vi "LVClass_SlopesPostProcessList Write SlopesPostProccessor  ptr create.vi"(8 "error in (no error)":errorcluster, 10 "Enum":T1, 11 "SlopesPostProcessorList in":refnum<class "SlopesPostProcessorList.lvclass">) -> (0 "error out":errorcluster, 3 "SlopesPostProcessorList out":refnum<class "SlopesPostProcessorList.lvclass">)   [LabVIEW 2020, in "SlopesPostProcessorList.lvclass"]
uses:
  SlopesPostProcessorList.lvclass
  Controls/Handle creation.ctl
  SlopesPostProcessorList.lvclass/SlopesPostProcessorList.ctl
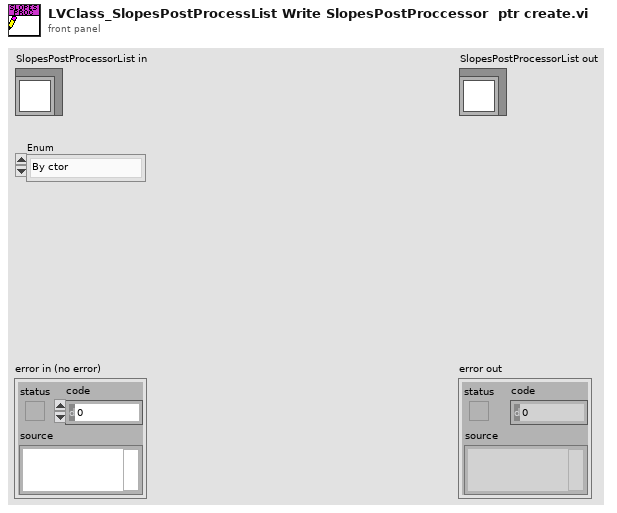
[diagram p1: front panel]
types:
  T1 = typedef "Handle creation.ctl" = enum16{"By ctor", "By write function"}
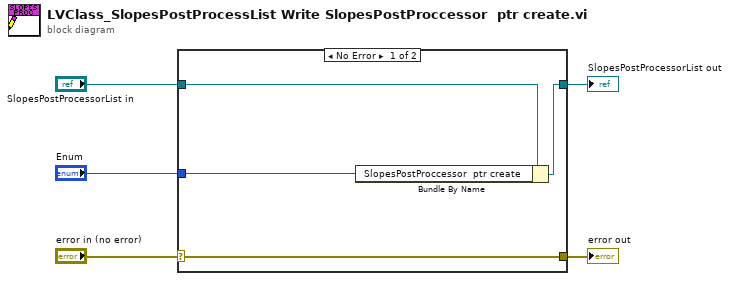
[diagram p0: block diagram]
diagram:
  n1 = case shown="No Error" "error in (no error)" {
    selector: "error in (no error)" -> [w9 w10]
    tunnel: [w9 w10] -> w4
    tunnel: [w7 w11] -> w2
    tunnel: "SlopesPostProcessorList in" -> [w8 w11]
    tunnel: "Enum" -> [w6 _]
    frame No Error {
      n2 = Bundle By Name(cluster=w8, "SlopesPostProccessor  ptr create"=w6) -> (w7:refnum<class "SlopesPostProcessorList.lvclass">)
    }
    frame Error {
    }
  }
  "error out" <- w4
  "SlopesPostProcessorList out" <- w2
